vi "BeeperTest2.vi"(0 "offset":dbl=79.1, 1 "Init":bool, 2 "sample rate":dbl=48000.0, 3 "number of samples":i32=512, 4 "Upper Cut-Off":dbl=5000.0, 5 "Lower Cut-Off":dbl=100.0, 7 "error in":errorcluster, 8 "VISA resource name":refnum<visa-resource-name>="COM10", 19 "Serial":string) -> (10 "N Harmonics":i32=4, 12 "Harmonic Array":T1(array[cluster])=[{"detected frequency"=43.09854330185955, "detected amplitude"=75.01663383722504, "detected phase (deg)"=-87.69885312031775}, {"detected frequency"=280.00916754679236, "detected amplitude"=60.43470449790236, "detected phase (deg)"=-73.50585748918513}, {"detected frequency"=592.6024100197471, "detected amplitude"=53.871301225844434, "detected phase (deg)"=258.4246806692645}, {"detected frequency"=1080.0344484932295, "detected amplitude"=49.52214668054196, "detected phase (deg)"=-50.198895521594864}], 13 "error out":errorcluster, 14 "PASS/FAIL 4":bool caption="PASS/FAIL", 15 "fundamental frequency":dbl=619.2259436114861 format="%.2p", 16 "fundamental amplitude":dbl=0.053981352584941814, 17 "fundamental dB output":dbl=53.74487524532033, 18 "THD":dbl=75.89686255102042 format="%.2p")   [LabVIEW 2014]
uses:
  <vilib>/express/express analysis/Spectral/Block/exnSpectralBlock spectral measurements peak poly.vi
  <vilib>/express/express analysis/Spectral/Block/exnSpectralBlock spectral measurements peak WFM.vi
  <vilib>/measure/matone.llb/Extract Multiple Tone Information 1 Chan.vi
  <vilib>/measure/matone.llb/Harmonic Distortion Analyzer 1 Chan.vi
  <vilib>/express/express analysis/Spectral/XNode/ExpressSpectralMeasurementsBlockNode.xnode
  <vilib>/measure/NI_MAPro.lvlib
panel:
  out "Beeper Time Domain AC":waveform(dbl)(graph)={"t0"=timestamp(3513633986.063842 s since 1904-01-01), "dt"=2.0833333101715314e-05, "Y"=array[500 elements], "attributes"=variant("NI_ChannelName"=variant(string "Sound Pressure (Extracted)"), "NI_ExpIsRelativeTime"=variant(bool FALSE), "NI_ExpStartTimeStamp"=variant(timestamp timestamp(3513633986.059675 s since 1904-01-01)), "NI_ExpTimeStamp"=variant(timestamp timestamp(3513633986.063842 s since 1904-01-01)), "NI_ExpXDimension"=variant(string "t"), "NI_OriginalChannelName"=variant(string "Sound Pressure"), "NI_UnitDescription"=variant(string "Pascals"), "NI_dBReference"=variant(dbl 2e-05))}
  out "FFT Mask":dynamicdata(graph)=[{"t0"=timestamp(0 s since 1904-01-01), "dt"=96.00000106729586, "Y"=array[250 elements]}, {"t0"=timestamp(0 s since 1904-01-01), "dt"=96.00000106729586, "Y"=[nan, 31.01897659055934, nan, 10.304743018244151, nan, 3.143345531596521, 3.739389040173816, 3.5002795002135985, 2.2963994395623084, 2.1181187702180746, 1.8836476164784564, 2.2259623676341866, 1.7934921207609553, 1.3719846482659466, 0.7451602376556167, 0.36297236489542156, 1.047605920313922, 0.4493831925428475, 0.42818504924119205, 0.2260045811295838, 0.45805557564447213, 0.5238226539579587, 0.4859327421596296, 0.11976281047355297, 0.6224799206857374, 0.5778447413555355, nan, nan, nan, nan, nan, nan, nan, nan, nan, nan, nan, 0.24200685544415995, 0.21862631469661264, 0.14751822621129868, 0.4947636594881805, 0.5964911450924486, 0.6309414533197579, 0.7235552883702737, 0.5481721786396152, 0.1776986736521948, 0.4701993437781902, 0.6234599416370945, 0.7626189439509773, 0.8488209029960562, 1.203455657248852, 1.7356432197560066, 1.2287772393120862, 0.48101254028153706, 0.30680529548526053, 0.1915095336616511, 0.3066097277355267, 0.6183026726148589, 0.46553971763340235, nan, nan, nan, nan, nan, nan, nan, nan, 0.21845835149121456, 0.2616386642156688, 0.26991518464539077, 0.30247639718566716, 0.2367124887765958, 0.05539020968555381, 0.26786560712917934, 0.19708158324139197, 0.1336448913956225, 0.0864738914835091, nan, 0.10080024271357395, 0.1697257799262496, 0.18213772310227624, 0.5357531131489985, 0.6271469432466881, 0.40297494159951436, 0.1443681647612314, 0.13255793714094447, nan, 0.10811213726306196, 0.07677764164778347, nan, nan, nan, nan, nan, nan, nan, nan, nan, nan, nan, nan, nan, nan, nan, nan, 0.3018103911479392, nan, nan, nan, nan, nan, nan, nan, nan, nan, nan, nan, nan, nan, nan, nan, nan, nan, nan, nan, nan, nan, nan, nan, nan, nan, nan, nan, nan, nan, nan, nan, nan, nan, nan, nan, nan, nan, nan, nan, nan, nan, nan, nan, nan, nan, nan, nan, nan, nan, nan, nan, nan, nan, nan, nan, nan, nan, nan, nan, nan, nan, nan, nan, nan, nan, nan, nan, nan, nan, nan, nan, nan, nan, nan, nan, nan, nan, nan, nan, nan, nan, nan, nan, nan, nan, nan, nan, nan, nan, nan, nan, nan, nan, nan, nan, nan, nan, nan, nan, nan, nan, nan, nan, nan, nan, nan, nan, nan, nan, nan, nan, nan, nan, nan, nan, nan, nan, nan, nan, nan, nan, nan, nan, nan, nan, nan, nan, nan, nan, nan, nan, nan, nan, nan, nan, nan, nan, nan, nan, nan, nan, nan, nan, nan], "attributes"=variant("NI_ChannelName"=variant(string "Failures"))}, {"t0"=timestamp(0 s since 1904-01-01), "dt"=96.00000106729586, "Y"=[10.0, 10.0, 10.0, 10.0, 10.0, 0.05, 0.05, 0.05, 0.05, 0.05, 0.05, 0.05, 0.05, 0.05, 0.05, 0.05, 0.05, 0.05, 0.05, 0.05, 0.05, 0.05, 0.05, 0.05, 0.05, 0.05, 18.404011072127098, 20.0, 20.0, 20.0, 20.0, 20.0, 20.0, 20.0, 20.0, 20.0, 20.0, 0.05, 0.05, 0.05, 0.05, 0.05, 0.05, 0.05, 0.05, 0.05, 0.05, 0.05, 0.05, 0.05, 0.05, 0.05, 0.05, 0.05, 0.05, 0.05, 0.05, 0.05, 0.05, 1.7160074934841216, 6.0, 6.0, 6.0, 6.0, 6.0, 6.0, 1.715991617458449, 0.05, 0.05, 0.05, 0.05, 0.05, 0.05, 0.05, 0.05, 0.05, 0.05, 0.05, 0.05, 0.05, 0.05, 0.05, 0.05, 0.05, 0.05, 0.05, 0.05, 0.05, 0.05, 0.05, 5.0, 5.0, 5.0, 5.0, 5.0, 5.0, 5.0, 3.847990061341082, 0.2, 0.2, 0.2, 0.2, 0.2, 0.2, 0.2, 0.2, 0.2, 0.2, 0.2, 0.2, 0.2, 0.2, 0.2, 0.2, 0.2, 0.2, 0.2, 0.2, 0.2, 0.2, 0.2, 0.2, 0.2, 0.2, 0.2, 0.2, 0.2, 0.2, 0.2, 0.2, 0.2, 0.2, 0.2, 0.2, 0.2, 0.2, 0.2, 0.2, 0.2, 0.2, 0.2, 0.2, 0.2, 0.2, 0.2, 0.2, 0.2, 0.2, 0.2, 0.2, 0.2, 0.2, 0.2, 0.2, 0.2, 0.2, 0.2, 0.2, 0.2, 0.2, 0.2, 0.2, 0.2, 0.2, 0.2, 0.2, 0.2, 0.2, 0.2, 0.2, 0.2, 0.2, 0.2, 0.2, 0.2, 0.2, 0.2, 0.2, 0.2, 0.2, 0.2, 0.2, 0.2, 0.2, 0.2, 0.2, 0.2, 0.2, 0.2, 0.2, 0.2, 0.2, 0.2, 0.2, 0.2, 0.2, 0.2, 0.2, 0.2, 0.2, 0.2, 0.2, 0.2, 0.2, 0.2, 0.2, 0.2, 0.2, 0.2, 0.2, 0.2, 0.2, 0.2, 0.2, 0.2, 0.2, 0.2, 0.2, 0.2, 0.2, 0.2, 0.2, 0.2, 0.2, 0.2, 0.2, 0.2, 0.2, 0.2, 0.2, 0.2, 0.2, 0.2, 0.2, 0.2, 0.2, 0.2, 0.2, 0.2, 0.2, 0.2, 0.2, 0.2, 0.2, 0.2, 0.2, 0.2, 0.2, 0.2, 0.2], "attributes"=variant("NI_ChannelName"=variant(string "Upper Limit"))}, {"t0"=timestamp(0 s since 1904-01-01), "dt"=96.00000106729586, "Y"=[0.0, 0.0, 0.0, 0.0, 0.0, 0.0, 0.0, 0.0, 0.0, 0.0, 0.0, 0.0, 0.0, 0.0, 0.0, 0.0, 0.0, 0.0, 0.0, 0.0, 0.0, 0.0, 0.0, 0.0, 0.0, 0.0, 0.0, 0.0, 0.0, 0.0, 0.0, 0.0, 0.0, 0.0, 0.0, 0.0, 0.0, 0.0, 0.0, 0.0, 0.0, 0.0, 0.0, 0.0, 0.0, 0.0, 0.0, 0.0, 0.0, 0.0, 0.0, 0.0, 0.0, 0.0, 0.0, 0.0, 0.0, 0.0, 0.0, 0.0, 0.0, 0.0, 0.0, 0.0, 0.0, 0.0, 0.0, 0.0, 0.0, 0.0, 0.0, 0.0, 0.0, 0.0, 0.0, 0.0, 0.0, 0.0, 0.0, 0.0, 0.0, 0.0, 0.0, 0.0, 0.0, 0.0, 0.0, 0.0, 0.0, 0.0, 0.0, 0.0, 0.0, 0.0, 0.0, 0.0, 0.0, 0.0, 0.0, 0.0, 0.0, 0.0, 0.0, 0.0, 0.0, 0.0, 0.0, 0.0, 0.0, 0.0, 0.0, 0.0, 0.0, 0.0, 0.0, 0.0, 0.0, 0.0, 0.0, 0.0, 0.0, 0.0, 0.0, 0.0, 0.0, 0.0, 0.0, 0.0, 0.0, 0.0, 0.0, 0.0, 0.0, 0.0, 0.0, 0.0, 0.0, 0.0, 0.0, 0.0, 0.0, 0.0, 0.0, 0.0, 0.0, 0.0, 0.0, 0.0, 0.0, 0.0, 0.0, 0.0, 0.0, 0.0, 0.0, 0.0, 0.0, 0.0, 0.0, 0.0, 0.0, 0.0, 0.0, 0.0, 0.0, 0.0, 0.0, 0.0, 0.0, 0.0, 0.0, 0.0, 0.0, 0.0, 0.0, 0.0, 0.0, 0.0, 0.0, 0.0, 0.0, 0.0, 0.0, 0.0, 0.0, 0.0, 0.0, 0.0, 0.0, 0.0, 0.0, 0.0, 0.0, 0.0, 0.0, 0.0, 0.0, 0.0, 0.0, 0.0, 0.0, 0.0, 0.0, 0.0, 0.0, 0.0, 0.0, 0.0, 0.0, 0.0, 0.0, 0.0, 0.0, 0.0, 0.0, 0.0, 0.0, 0.0, 0.0, 0.0, 0.0, 0.0, 0.0, 0.0, 0.0, 0.0, 0.0, 0.0, 0.0, 0.0, 0.0, 0.0, 0.0, 0.0, 0.0, 0.0, 0.0, 0.0, 0.0, 0.0, 0.0, 0.0, 0.0, 0.0, 0.0, 0.0, 0.0, 0.0, 0.0, 0.0], "attributes"=variant("NI_ChannelName"=variant(string "Lower Limit"))}]
  out "number of cycles \nbefore sample acquisition":i32=4
  out "Beeper Time Domain":waveform(dbl)(graph)={"t0"=timestamp(3513633986.059675 s since 1904-01-01), "dt"=2.0833333101715314e-05, "Y"=array[700 elements], "attributes"=variant("NI_ChannelName"=variant(string "Sound Pressure (Trigger)"), "NI_OriginalChannelName"=variant(string "Sound Pressure"), "NI_UnitDescription"=variant(string "Pascals"), "NI_dBReference"=variant(dbl 2e-05))}
  out "FFT Peak":cluster{"f0":dbl, "df":dbl, "magnitude":dbl[]}(graph)={"f0"=0.0, "df"=96.00000106729586, "magnitude"=[0.05841699805737301, 0.3921488823079563, 0.10740215441957349, 0.13027488012950889, 0.05897325153761291, 0.039738881562535036, 0.04727419772659692, 0.044251321115216166, 0.0290315984773996, 0.026777734136764535, 0.023813497047768098, 0.028141117163516898, 0.0226737309830715, 0.017344938663286305, 0.009420483409046988, 0.004588778317261967, 0.01324406978905085, 0.005681203445548009, 0.005413211747676259, 0.0028572007728139546, 0.005790841664279041, 0.006622283867989365, 0.006143271076607202, 0.0015140684004241844, 0.007869531234965076, 0.007305243253546594, 0.007816641292822871, 0.013068314186396552, 0.0055501020584829246, 0.0017735753926981393, 0.006585325974213076, 0.009704427856766389, 0.00988465202435985, 0.007178510878884607, 0.006247956709046263, 0.005938930967489451, 0.00544646013804486, 0.003059505125716308, 0.0027639230682251917, 0.0018649586120265322, 0.0062549135207102475, 0.0075409752856188195, 0.007976503834636637, 0.009147348778385257, 0.0069301160384275, 0.002246506620128885, 0.005944365913757146, 0.00788192088036782, 0.009641200302793645, 0.01073098486720678, 0.015214357234498762, 0.021942392158735863, 0.015534478373098437, 0.0060810687772634275, 0.003878701586412902, 0.002421106620248434, 0.0038762291749118425, 0.007816721524840189, 0.005885457871471585, 0.004254510137483866, 0.005132401757676973, 0.0014485965182118195, 0.0015551016847785667, 0.0012366908313783086, 0.0006871258848273028, 0.0013175598690578284, 0.002301837450156382, 0.002761799639585519, 0.003307694869983171, 0.003412328503734397, 0.003823974679970508, 0.0029925725509051303, 0.0007002554953925894, 0.0033864172835547327, 0.002491549724922781, 0.0016895687913479457, 0.001093222395493162, 0.0005927680116288617, 0.001274339351625461, 0.00214571150349241, 0.0023026260822032398, 0.006773111417812877, 0.007928532784408193, 0.005094499893799171, 0.001825134826311396, 0.0016758272710612448, 0.0005555368838957886, 0.0013667779679274585, 0.0009706402231072501, 0.0005580234209451316, 0.0008681098303268095, 0.0009111694287276712, 0.0014728871200535188, 0.0006726034187867432, 0.0017782118448832719, 0.0038987494875321513, 0.0028958627651206555, 0.0014638868420973517, 0.0017475247459314265, 0.000655951249486841, 0.00047203703103055895, 0.001396107920432402, 0.0009433336292884466, 0.0009058693538594409, 0.0010841498175750209, 0.0038155548817691435, 0.0023744034728087294, 0.0014055917542342277, 0.0024286210868487202, 0.0015852392736733494, 0.00044056678177576184, 0.00018680318618003955, 0.0005637898620662507, 0.0014960592172313747, 0.0018328583686046977, 0.001389720637130814, 0.0012265473860588146, 0.0008491191887753687, 0.0006869289829724649, 0.0020629716458314836, 0.0011552408858355068, 0.002305508068488998, 0.002399934994577758, 0.0009489091930337609, 0.00038486577776829846, 0.0014247053833866756, 0.0018373008598047437, 0.0010600331707726108, 0.0010329784349807022, 0.0011489617801774207, 0.0015477359984200668, 0.0015081916305745987, 0.0015308096481146244, 0.0009779694077318589, 0.0018283769747305131, 0.001524189603900281, 0.00047955077805208226, 0.002334268047423524, 0.001744035270866101, 0.0015614232735818188, 0.0021726567115095846, 0.0009952194750947388, 0.0004503168106901299, 0.0002770545327596492, 0.001232822475506275, 0.0016243830037005063, 0.001211798767916498, 0.0005664080397552238, 0.0009918453725469485, 0.0010480721352134925, 0.0009699922295284301, 0.00042674899928002593, 0.0002514816331496148, 0.0005078229983380667, 0.0005730998052512297, 0.0004160192662989664, 0.0001465907271066361, 0.0005467702203761605, 0.0007346759251726099, 0.000637954457286619, 0.0003341456024715272, 0.00019434421873787882, 0.00021795005298427253, 0.00016152799658884998, 0.0003511394983805079, 0.0004193055523946284, 0.00048689823480517594, 0.00016590055411030153, 0.0002700922790323925, 0.00040968766873039923, 0.0002601085972299943, 0.0002560113888270391, 0.0004033390262031513, 0.0003782610923996281, 0.0002330461012279771, 0.00026864452569483235, 0.0001890611915922127, 4.723348067783229e-05, 6.311295838691933e-05, 0.00023715780085499288, 0.0004398644149748958, 0.00034839330441722814, 0.00019227448525304031, 0.0001095314856252162, 6.47024173745757e-05, 0.00010758127940211323, 4.9140680149569146e-05, 0.00016653612582793862, 0.00022015444675685923, 0.00012859870835915394, 9.597378501753013e-05, 0.0001372810430656223, 0.00012650997324302783, 5.905341481274702e-05, 0.00020847958584877937, 0.00023063701601928343, 0.00023319861900986105, 0.000266621422660342, 0.0002752855605550971, 0.00021952307680459283, 2.3369619567350572e-05, 3.732150373027298e-05, 0.00015761650633764005, 4.351757546774082e-05, 0.00018216586713419683, 0.00017550799719793386, 0.00019337701047406349, 9.32698230280218e-05, 0.00022886688837124987, 0.00025841334470113367, 0.000398921298413115, 0.00031437860653351295, 0.000124896924497091, 0.00016823626930025602, 0.00014767493536391673, 9.369998569294706e-05, 0.0002621924542756944, 0.0002527592347092638, 0.00016024556713666697, 6.995096765792457e-05, 9.899402500774186e-05, 0.00014619791276626346, 0.00012117176272181464, 7.638718602691197e-05, 4.997726711562398e-05, 5.030696429353662e-05, 7.614853950100376e-05, 4.984029628072504e-05, 3.0290957222420546e-05, 4.6385651681067275e-05, 0.00011764282956353552, 0.0001546374332542939, 8.879599686459558e-05, 1.1562667563243625e-05, 2.2785403926692664e-05, 3.443607170173395e-05, 5.404102870156626e-05, 2.814447798324508e-05, 1.4765059373329104e-05, 2.5615884562841033e-05, 2.5908642346403393e-05, 1.6836428773156306e-05, 2.4603925330282385e-06, 1.64454345169931e-05, 8.162172043887631e-06, 8.163267196629857e-06, 1.5554184235528123e-05, 4.067362866266299e-06, 3.4371719107197144e-06, 2.8004576585125405e-06]}
  # "Trigger at 0.8"
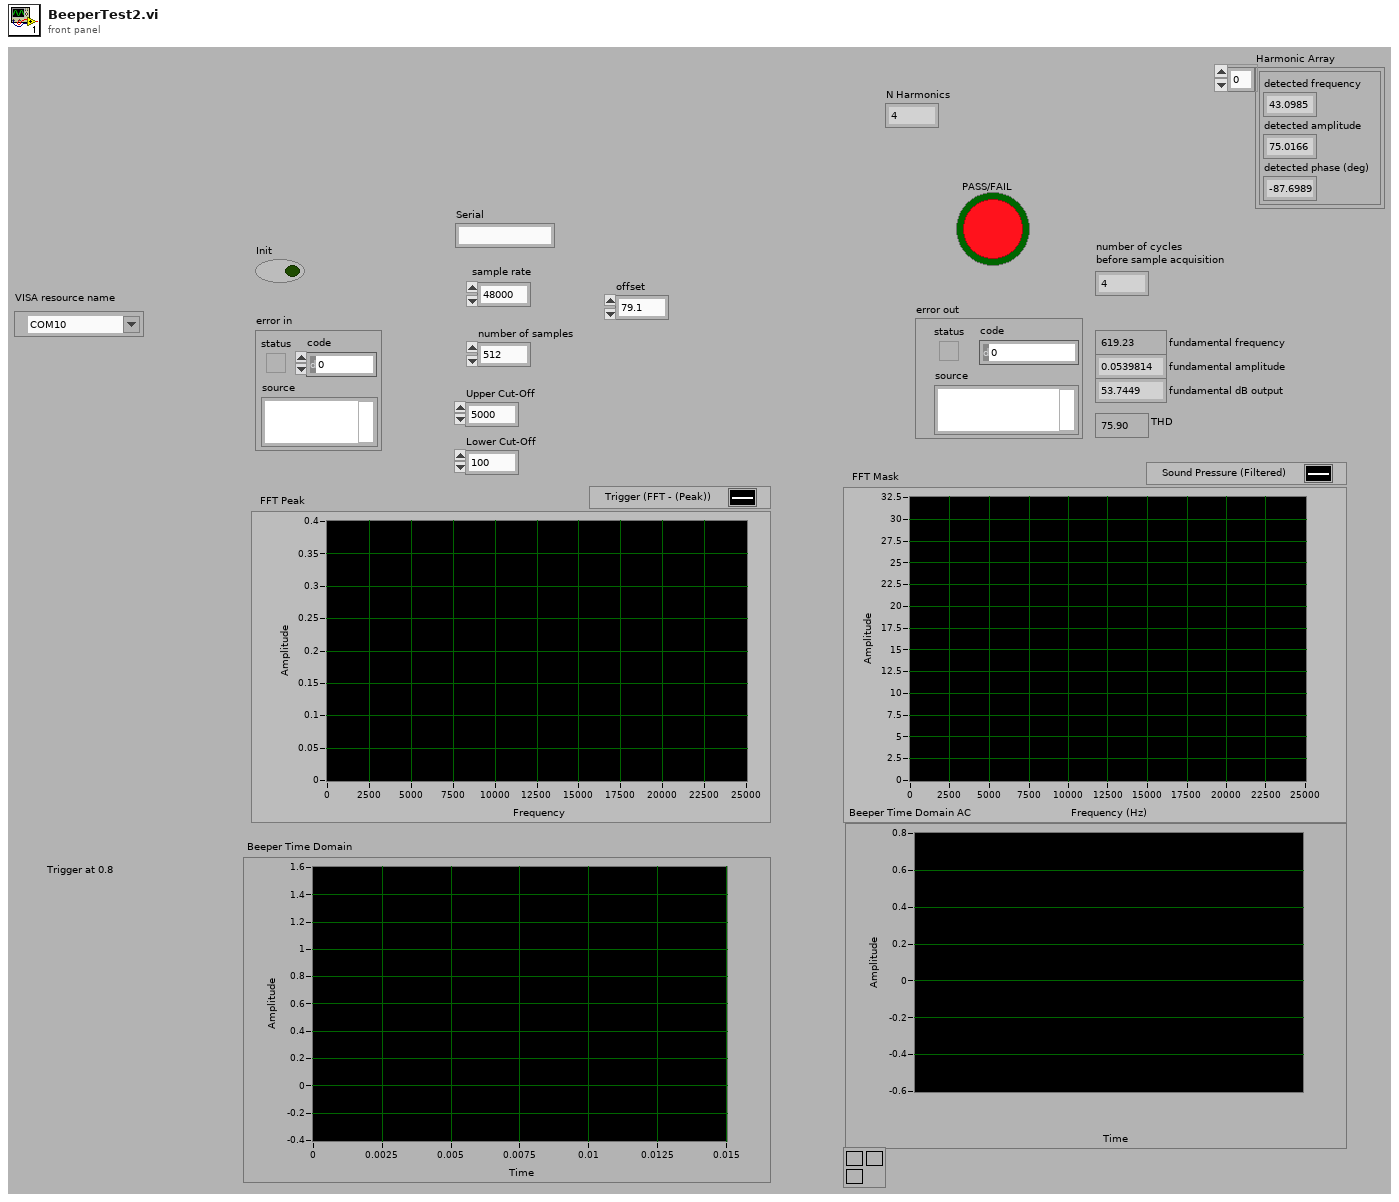
[diagram p1: front panel]
types:
  T1 = cluster{"detected frequency":dbl, "detected amplitude":dbl, "detected phase (deg)":dbl}[]
  T2 = enum16{"Enter FAT", "Beeper Control", "LED Off", "LED On", "Image Mode", "Start Session", "Stop Session", "Change Buadrate", "Auto Exposure", "Set Manual Exposure", "Read BT Address", "Store BT Address", "Pairing Command", "Query Paired Address", "Pairing Status", "Un-Pairing", "Set Illumination", "Trigger", "Set Defaults", "Imager Time To Decode Test", "Battery Off", "Battery Charge Control", "Read Battery Voltage", "Read Battery Temperature", "Software Version", "StoreFeatureSet", "ReadFeatureSet", "Store Model Number", "Read Model Number", "Store Manufacturing Date", "Read Manufacturing Date", "Store Service Date", "Read Service Date", "Store Serial Number", "Read Serial Number", "Exit FAT", "Read GUID", "Cable Auto ID", "Store RSM 627", "Read RSM 627", "Hall Effect switch", "Store GUID ", "ParamSend", "General", "General-Response", "RSM Init", "RSM EnterFAT", "RSM - SE4500 - Peek PRISM Register GENERIC command", "RSM - SE4500 - Poke PRISM Register GENERIC command", "RSM - SE4500 - GENERIC command", "RSM - SE4500 - GetPDM Calibration", "RSM - SE4500 - SetPDM Calibration", "Get Object Sensor Value", "Store Object Sensor Calibration Value", "Read Object Sensor Calibration Value", "RSM - SE4500 - GetPDM-Z Calibration", "RSM - SE4500 - SetPDM-Z Calibration"}
  T3 = cluster{"averaging mode":u16, "weighting mode":u16, "number of averages":u32}
  T4 = cluster{"dB On (F)":bool, "unwrap phase (F)":bool, "convert to degree (F)":bool}
  T5 = enum32{"none", "input signal", "detected signal", "residual signal"}
  T6 = cluster{"approx freq. (optional)":dbl, "search (+/- % of Fsampl.)":dbl}
  T7 = enum16{"none", "input signal", "fundamental signal", "residual signal", "harmonics only", "noise and spurs"}
  T8 = cluster{"detected frequency":dbl, "detected amplitude":dbl, "detected phase (deg)":dbl}
  T9 = cluster{"detected frequency":dbl, dbl, "detected phase (deg)":dbl}
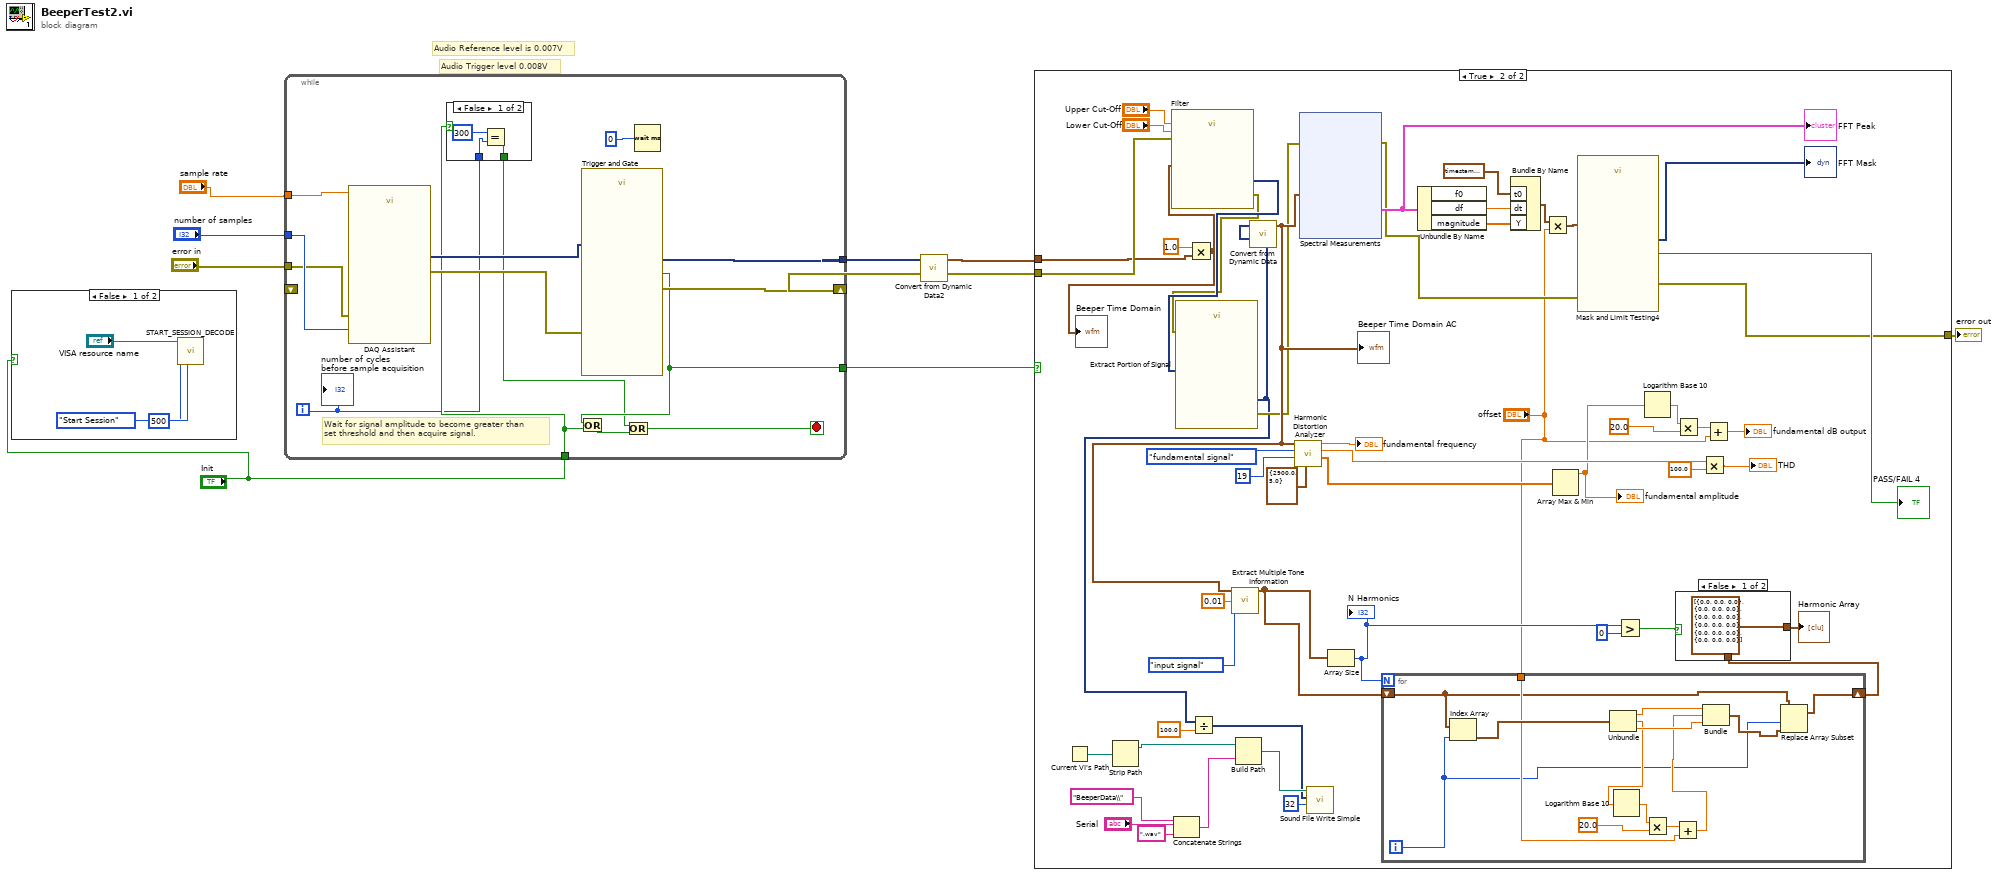
[diagram p0: block diagram]
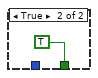
[diagram p3: hidden frame]
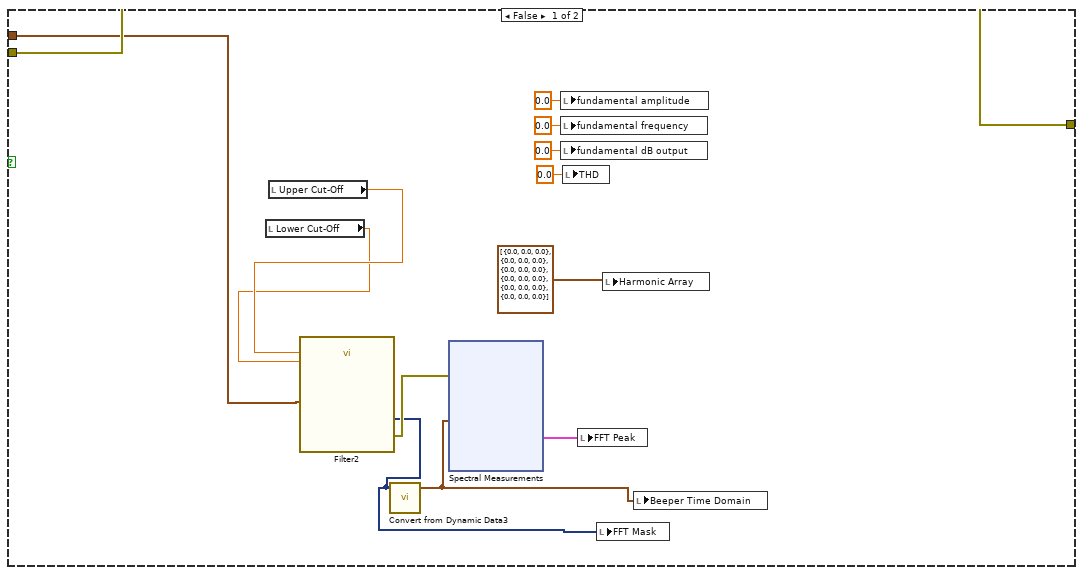
[diagram p4: hidden frame]
diagram:
  # "Audio Trigger level 0.008V"
  # "Audio Reference level is 0.007V"
  n1 = case shown="False" "Init" {
    frame False {
      n2 = call "START_SESSION_DECODE.vi"("MIMIC HOST COMMAND"=T2."Start Session", "wait (ms)"=u32 500, "VISA resource name"="VISA resource name") -> ()  [unwired: 6 in, 3 out]
    }
    frame True {
    }
  }
  n3 = while {
    tunnel: [w18] -> w6
    shift-right: [w24] -> w5
    shift-left: _ -> [_]
    tunnel: [w26] -> w4
    tunnel: "sample rate" -> [w22]
    tunnel: "number of samples" -> [w21]
    tunnel: "error in" -> [w19]
    tunnel: "Init" -> [w15]
    i -> [w13]
    stop <- w16 stop-if-true
    # "Wait for signal amplitude to become greater than\nset threshold and then acquire signal."
    n4 = call "DAQ Assistant"("rate"=w22, "number of samples"=w21, "error in"=w19) -> ("data"=w23:dynamicdata, "error out"=w20:errorcluster)  [unwired: 13 in, 2 out]
    n5 = case shown="False" w15 {
      tunnel: w13 -> [w29 _]
      tunnel: [w27 TRUE] -> w14
      frame False {
        n6 = Equal?(x=300, y=w29) -> (x = y?=w27:bool)
      }
      frame True {
      }
    }
    n7 = call "Trigger and Gate"("error in (no error)"=w20, "Signals"=w23) -> ("error out"=w24:errorcluster, "Triggered Signals"=w26:dynamicdata, "Data Available"=w18:bool)  [unwired: 6 in, 1 out]
    n8 = Or(x=w18, y=w15) -> (x .or. y?=w17:bool)
    n9 = Or(x=w14, y=w17) -> (x .or. y?=w16:bool)
    n10 = Wait (ms)(milliseconds to wait=u32 0) -> ()  [unwired: 1 out]
    "number of cycles \nbefore sample acquisition" <- w13
  }
  n11 = call "Convert from Dynamic Data2"("Dynamic Data Type"=w4) -> ("Waveform"=w7:waveform(dbl))  [unwired: 3 in]
  n12 = case shown="True" w6 {
    tunnel: w7 -> [w36 w102]
    tunnel: w5 -> [w43 w103]
    tunnel: [w43 w104] -> w2
    frame False {
      n13 = local read "Lower Cut-Off"() -> (w34:dbl)
      n14 = local read "Upper Cut-Off"() -> (w35:dbl)
      n15 = call "Filter2"("Lower Cut-Off"=w34, "Upper Cut-Off"=w35, "Signal"=w36) -> ("error out"=w37:errorcluster, "Filtered Signal"=w32:dynamicdata)  [unwired: 7 in]
      n16 = call "Convert from Dynamic Data3"("Dynamic Data Type"=w32) -> ("Waveform"=w33:waveform(dbl))  [unwired: 3 in]
      n17 = xnode "Spectral Measurements"("Signals"=w33, "error in (no error)"=w37) -> ("FFT - (Peak)"=w31:cluster{"f0":dbl, "df":dbl, "magnitude":dbl[]})  [unwired: 2 out]
      n18 = local write "fundamental amplitude"(0.0 ("fundamental amplitude")) -> ()
      n19 = local write "fundamental frequency"(0.0 ("fundamental frequency")) -> ()
      n20 = local write "fundamental dB output"(0.0 ("fundamental dB output")) -> ()
      n21 = local write "THD"(0.0 ("THD")) -> ()
      n22 = local write "FFT Peak"(w31) -> ()
      n23 = local write "FFT Mask"(w32) -> ()
      n24 = local write "Harmonic Array"(T1 [{"detected frequency"=0.0, "detected amplitude"=0.0, "detected phase (deg)"=0.0}, {"detected frequency"=0.0, "detected amplitude"=0.0, "detected phase (deg)"=0.0}, {"detected frequency"=0.0, "detected amplitude"=0.0, "detected phase (deg)"=0.0}, {"detected frequency"=0.0, "detected amplitude"=0.0, "detected phase (deg)"=0.0}, {"detected frequency"=0.0, "detected amplitude"=0.0, "detected phase (deg)"=0.0}, {"detected frequency"=0.0, "detected amplitude"=0.0, "detected phase (deg)"=0.0}] ("multiple tone information")) -> ()
      n25 = local write "Beeper Time Domain"(w33) -> ()
    }
    frame True {
      n26 = Current VI's Path() -> (path=w62:path)
      n27 = Strip Path(path=w62) -> (stripped path=w61:path)  [unwired: 1 out]
      n28 = Concatenate Strings("BeeperData\\" ("string"), "Serial", ".wav" ("string")) -> (w66:string)
      n29 = Multiply(x=1.0, y=w102) -> (x*y=w100:waveform(dbl))
      "Beeper Time Domain" <- w100
      n30 = call "Filter"("error in (no error)"=w103, "Lower Cut-Off"="Lower Cut-Off", "Upper Cut-Off"="Upper Cut-Off", "Signal"=w100) -> ("error out"=w57:errorcluster, "Filtered Signal"=w68:dynamicdata)  [unwired: 6 in]
      n31 = call "Extract Portion of Signal"("error in (no error)"=w57, "Signals"=w68) -> ("error out"=w58:errorcluster, "Section"=w56:dynamicdata)  [unwired: 8 in]
      n32 = Divide(x=w56, y=100.0) -> (x/y=w54:dynamicdata)
      n33 = Build Path(base path=w61, name or relative path=w66) -> (appended path=w60:path)
      n34 = call "Convert from Dynamic Data"("Dynamic Data Type"=w56) -> ("Waveform"=w59:waveform(dbl))  [unwired: 3 in]
      "Beeper Time Domain AC" <- w59
      n35 = call-poly <vilib>:"Extract Multiple Tone Information.vi"("time signal in"=w59, "export mode"=T5."input signal", "threshold"=0.01) -> ("multiple tone information"=w76:T1)  [unwired: 10 in, 2 out]
      n36 = call-poly <vilib>:"Harmonic Distortion Analyzer.vi"("advanced search"=T6 {"approx freq. (optional)"=2900.0, "search (+/- % of Fsampl.)"=5.0}, "highest harmonic"=19, "export mode"=T7."fundamental signal" ("export signals"), "signal in"=w59) -> ("components level"=w93:dbl[], "THD"=w83:dbl, "detected fundamental frequency"=→"fundamental frequency":dbl)  [unwired: 2 in, 3 out]
      n37 = xnode "Spectral Measurements"("Signals"=w59, "error in (no error)"=w58) -> ("FFT - (Peak)"=w99:cluster{"f0":dbl, "df":dbl, "magnitude":dbl[]}, "error out"=w79:errorcluster)  [unwired: 1 out]
      "FFT Peak" <- w99
      n38 = call <vilib>:"Sound File Write Simple.vi"("bits per sample"=32, "data"=w54, "path"=w60) -> ()  [unwired: 7 in, 2 out]
      n39 = Array Size(array=w76) -> (size(s)=w75:i32)
      "N Harmonics" <- w75
      n40 = for {
        N: w75 -> [_]
        tunnel: "offset" -> [w112]
        shift-right: [w110] -> w72
        shift-left: w76 -> [w109]
        i -> [w111]
        n41 = Index Array(array=w109, index=w111) -> (element=w121:T8)
        n42 = Unbundle(w121) -> ("detected frequency"=w120:dbl, "detected amplitude"=w114:dbl, "detected phase (deg)"=w119:dbl)
        n43 = Logarithm Base 10(1:w114) -> (0:w117:dbl)
        n44 = Multiply(x=w117, y=20.0) -> (x*y=w115:dbl)
        n45 = Add(x=w115, y=w112) -> (x+y=w113:dbl)
        n46 = Bundle("detected frequency"=w120, w113, "detected phase (deg)"=w119) -> (w118:T9)  [unwired: 1 in]
        n47 = Replace Array Subset(array=w109, new element=w118, index=w111) -> (w110:T1)
      }
      n48 = Unbundle By Name(w99) -> ("df"=w98:dbl, "magnitude"=w97:dbl[])  [unwired: 1 out]
      n49 = Bundle By Name("t0"=timestamp(0 s since 1904-01-01), "dt"=w98, "Y"=w97) -> (w80:waveform(dbl))  [unwired: 1 in]
      n50 = Multiply(x=w80, y="offset") -> (x*y=w81:waveform(dbl))
      n51 = Array Max & Min(array=w93) -> (max value=w82:dbl)  [unwired: 3 out]
      "fundamental amplitude" <- w82
      n52 = call "Mask and Limit Testing4"("error in"=w79, "Signals"=w81) -> ("error out"=w104:errorcluster, "Passed"=→"PASS/FAIL 4":bool, "Tested Signals"=→"FFT Mask":dynamicdata)  [unwired: 6 in, 1 out]
      n53 = Greater?(x=w75, y=0) -> (0:w73:bool)
      n54 = Logarithm Base 10(1:w82) -> (0:w92:dbl)
      n55 = Multiply(x=w92, y=20.0) -> (x*y=w90:dbl)
      n56 = case shown="False" w73 {
        tunnel: w72 -> [_ w108]
        tunnel: [T1 [{"detected frequency"=0.0, "detected amplitude"=0.0, "detected phase (deg)"=0.0}, {"detected frequency"=0.0, "detected amplitude"=0.0, "detected phase (deg)"=0.0}, {"detected frequency"=0.0, "detected amplitude"=0.0, "detected phase (deg)"=0.0}, {"detected frequency"=0.0, "detected amplitude"=0.0, "detected phase (deg)"=0.0}, {"detected frequency"=0.0, "detected amplitude"=0.0, "detected phase (deg)"=0.0}, {"detected frequency"=0.0, "detected amplitude"=0.0, "detected phase (deg)"=0.0}] ("multiple tone information") w108] -> w69
        frame False {
        }
        frame True {
        }
      }
      "Harmonic Array" <- w69
      n57 = Multiply(x=w83, y=100.0) -> (x*y=→"THD":dbl)
      n58 = Add(x=w90, y="offset") -> (x+y=→"fundamental dB output":dbl)
    }
  }
  "error out" <- w2
